vi "ADIS16470 Read Multiple Registers.vi"(8 "error in (no error)":errorcluster, 10 "Registers":T3[](array[typedef]) items=["Reserved", "_Reserved", "DIAG_STAT", "_DIAG_STAT", "X_GYRO_LOW", "_X_GYRO_LOW", "X_GYRO_OUT", "_X_GYRO_OUT", "Y_GYRO_LOW", "_Y_GYRO_LOW", ""], 11 "SPIDevRef":T1) -> (0 "error out":errorcluster, 3 "Values":i16[](array[numeric]))   [LabVIEW 2018]
uses:
  Typedef/ADIS16470 Register.ctl
  <vilib>/Rock Robotics/WPI/SPI/WPI_SPIDevRef.ctl
  <vilib>/Rock Robotics/SystemInterfaces/spilib/spi_bus.ctl
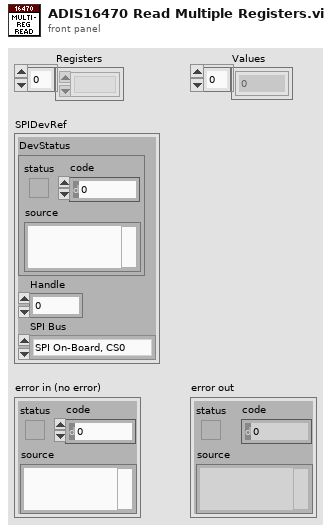
[diagram p1: front panel]
types:
  T1 = typedef "WPI_SPIDevRef.ctl" = cluster{"DevStatus":errorcluster, "Handle":i32, "SPI Bus":T2}
  T2 = typedef "spi_bus.ctl" = enum16{"SPI On-Board, CS0", "SPI On-Board, CS1", "SPI On-Board, CS2", "SPI On-Board, CS3", "SPI MXP", "Invalid"}
  T3 = typedef "ADIS16470 Register.ctl" = u32
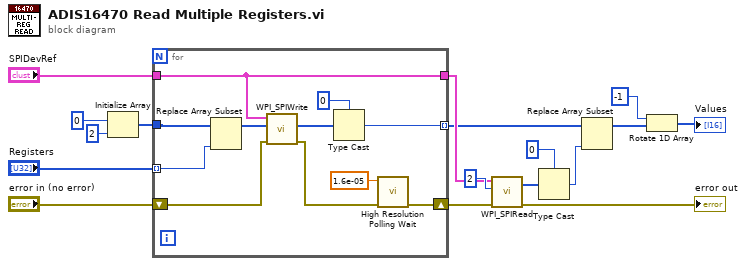
[diagram p0: block diagram]
diagram:
  n1 = Initialize Array(u8 0 ("element"), 2 ("dimension size")) -> (w7:u8[])
  n2 = for {
    tunnel: w7 -> [w24]
    tunnel: "Registers" -> [w25] mode=indexing
    tunnel: "SPIDevRef" -> [w21]
    shift-right: [w19] -> w4
    shift-left: "error in (no error)" -> [w23]
    tunnel: [w22] -> w2 mode=indexing
    tunnel: [w21] -> w3
    n3 = Replace Array Subset(array=w24, new element=w25) -> (w26:u8[])  [unwired: 1 in]
    n4 = call <vilib>:"WPI_SPIWrite.vi"("error in (no error)"=w23, "Data To Send"=w26, "SPIDevRef"=w21) -> ("error out"=w20:errorcluster, "Received Data"=w27:u8[])  [unwired: 7 out]
    n5 = Type Cast(type=i16 0, x=w27) -> (*(type *) &x=w22:i16)
    n6 = call <vilib>:"High Resolution Polling Wait.vi"("error in (no error)"=w20, "seconds to wait"=1.6e-05) -> ("error out"=w19:errorcluster)  [unwired: 9 in]
  }
  n7 = call <vilib>:"WPI_SPIRead.vi"("error in (no error)"=w4, "Num to Read"=2, "SPIDevRef"=w3) -> ("error out"=→"error out":errorcluster, "Received Data"=w13:u8[])  [unwired: 6 in, 1 out]
  n8 = Type Cast(type=i16 0, x=w13) -> (*(type *) &x=w12:i16)
  n9 = Replace Array Subset(array=w2, new element=w12) -> (w11:i16[])  [unwired: 1 in]
  n10 = Rotate 1D Array(1:w11, 2:-1 ("n")) -> (0:→"Values":i16[])
